vi "Sub_GaussFunctionCalc.vi"(1 "Mean":dbl, 2 "Standard deviation":dbl, 3 "Input":dbl) -> (0 "Gaussian output":dbl)   [LabVIEW 2021]
panel:
  out "XY Graph":cluster{dbl[], dbl[]}(graph)
  # "Inputs:"
  # "Outputs:"
  # "Required:"
  # "Debug purposes only (requires changes in diagram)"
  # "Optional:"
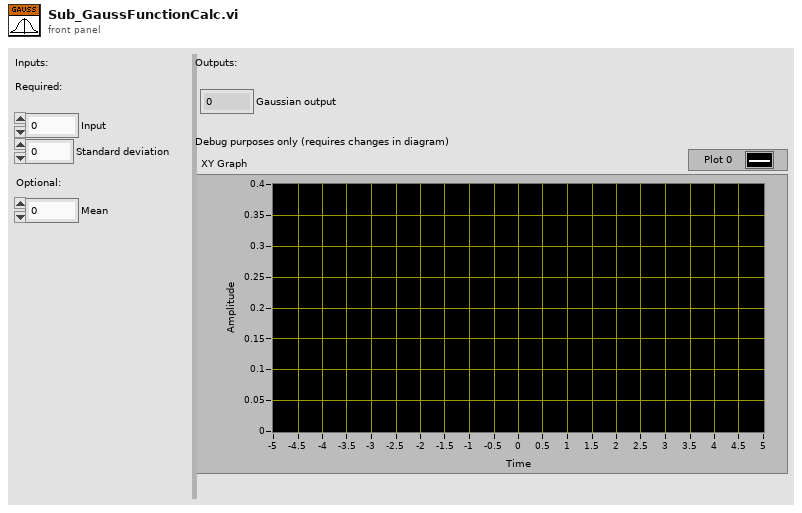
[diagram p1: front panel]
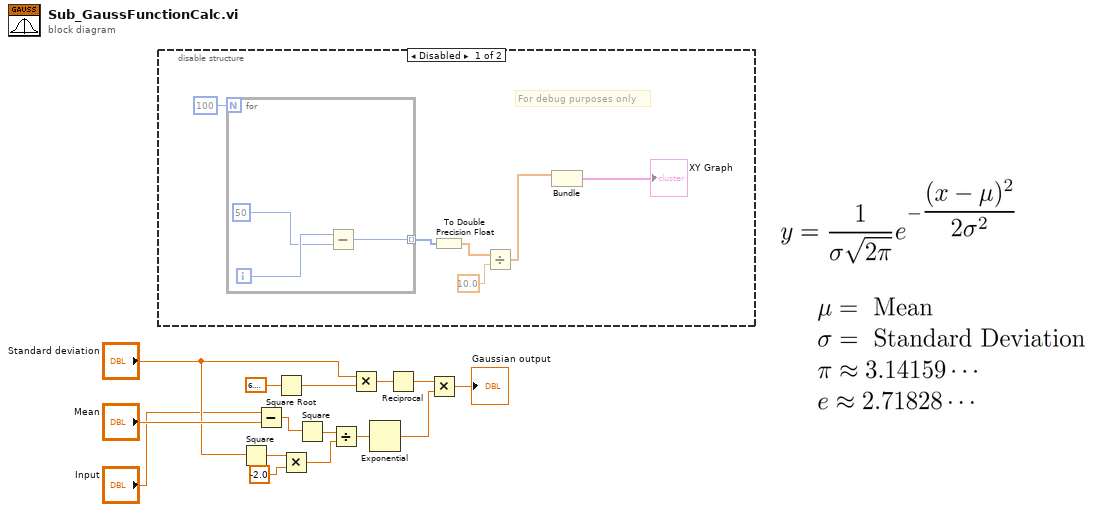
[diagram p0: block diagram]
diagram:
  n1 = disable-structure shown="Disabled" {
    frame Disabled {
      # "For debug purposes only"
      n2 = for {
        N: 100 -> [_]
        tunnel: [w22] -> w21 mode=indexing
        i -> [w24]
        n3 = Subtract(x=w24, y=50) -> (x-y=w22:i32)
      }
      n4 = To Double Precision Float(number=w21) -> (double precision float=w20:dbl[])
      n5 = Divide(x=w20, y=10.0) -> (x/y=w18:dbl[])
      n6 = Bundle(w18) -> (→"XY Graph":cluster{dbl[], void})  [unwired: 2 in]
    }
    frame Enabled {
    }
  }
  n7 = Square(x="Standard deviation") -> (x^2=w9:dbl)
  n8 = Subtract(x="Input", y="Mean") -> (x-y=w6:dbl)
  n9 = Square Root(x=6.283185307179586) -> (sqrt(x)=w11:dbl)
  n10 = Multiply(x=w9, y=-2.0) -> (x*y=w7:dbl)
  n11 = Square(x=w6) -> (x^2=w10:dbl)
  n12 = Divide(x=w10, y=w7) -> (x/y=w4:dbl)
  n13 = Multiply(x="Standard deviation", y=w11) -> (x*y=w13:dbl)
  n14 = Exponential(1:w4) -> (0:w14:dbl)
  n15 = Reciprocal(x=w13) -> (1/x=w15:dbl)
  n16 = Multiply(x=w15, y=w14) -> (x*y=→"Gaussian output":dbl)
